vi "Sub_Generator_control.vi"(0 "Amplitude":dbl=4.5 min=1.0 max=5.0 step=0.2 format="%#.1f") -> (1 "Generator signal type 2":string(combo), 2 "Frequency 2":dbl=10.0 min=10.0 max=200.0 step=5.0 format="%#.1g", 3 "Amplitude 2":dbl=1.0 min=0.2 max=2.0 step=0.2 format="%#.1g")   [LabVIEW 2020]
panel:
  in  "Back":bool
  in  "Frequency":dbl=10.0 min=5.0 max=100.0 step=5.0 format="%#.0f"
  in  "Generator signal type":string(combo)="Saw"
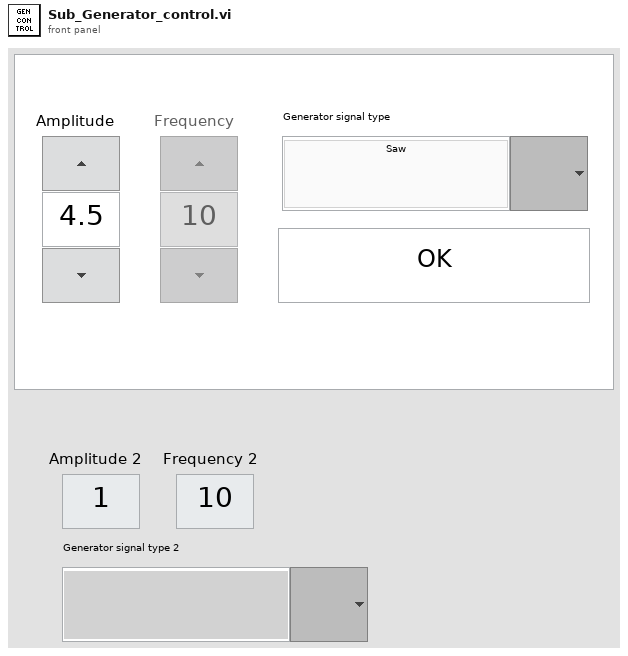
[diagram p1: front panel]
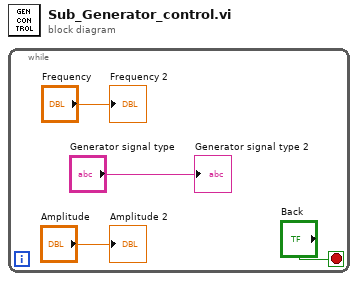
[diagram p0: block diagram]
diagram:
  n1 = while {
    stop <- "Back" stop-if-true
    "Generator signal type 2" <- "Generator signal type"
    "Frequency 2" <- "Frequency"
    "Amplitude 2" <- "Amplitude"
  }
